vi "手动启动选择对话框.vi"() -> (2 "确定":bool, 3 "输出簇":T1)   [LabVIEW 2016, in "PLC.lvlib"]
uses:
  PLC.lvlib
panel:
  in  "总磷":bool
  in  "测试模式":enum16{"正常测试", "集成干预"}(ring)
  in  "CODCr":bool
  in  "总氮":bool
  in  "氨氮":bool
  in  "CODmn":bool
  in  "多参数":bool
  in  "取消":bool
  in  "确定":bool
  # "请选择启动参数"
  # "请选择启动模式："
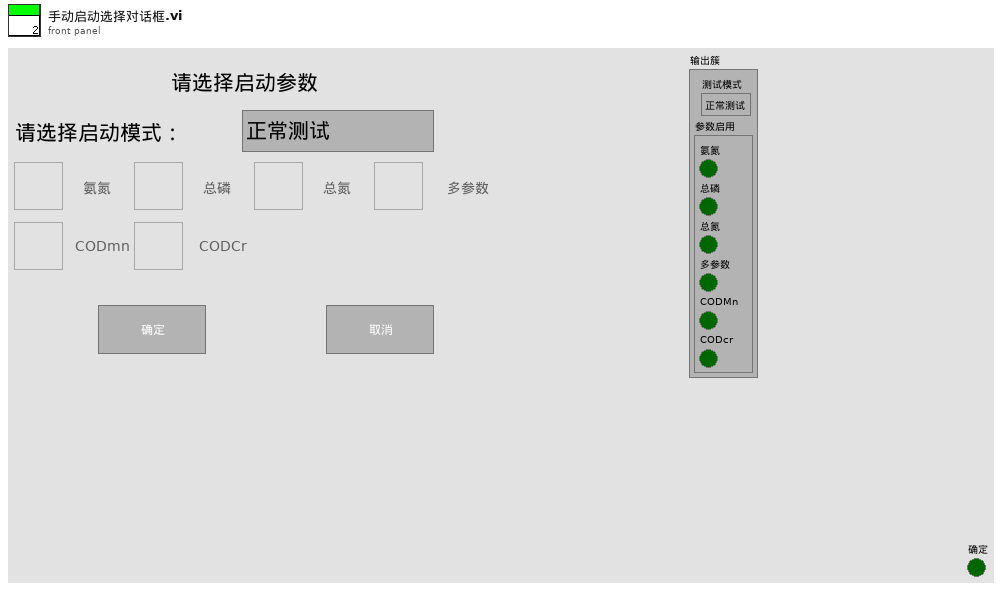
[diagram p1: front panel]
types:
  T1 = cluster{"测试模式":enum16{"正常测试", "集成干预"}, "参数启用":cluster{"氨氮":bool, "总磷":bool, "总氮":bool, "多参数":bool, "CODMn":bool, "CODcr":bool}}
  T2 = enum8{"Enabled", "Disabled", "Disabled and Grayed Out"}
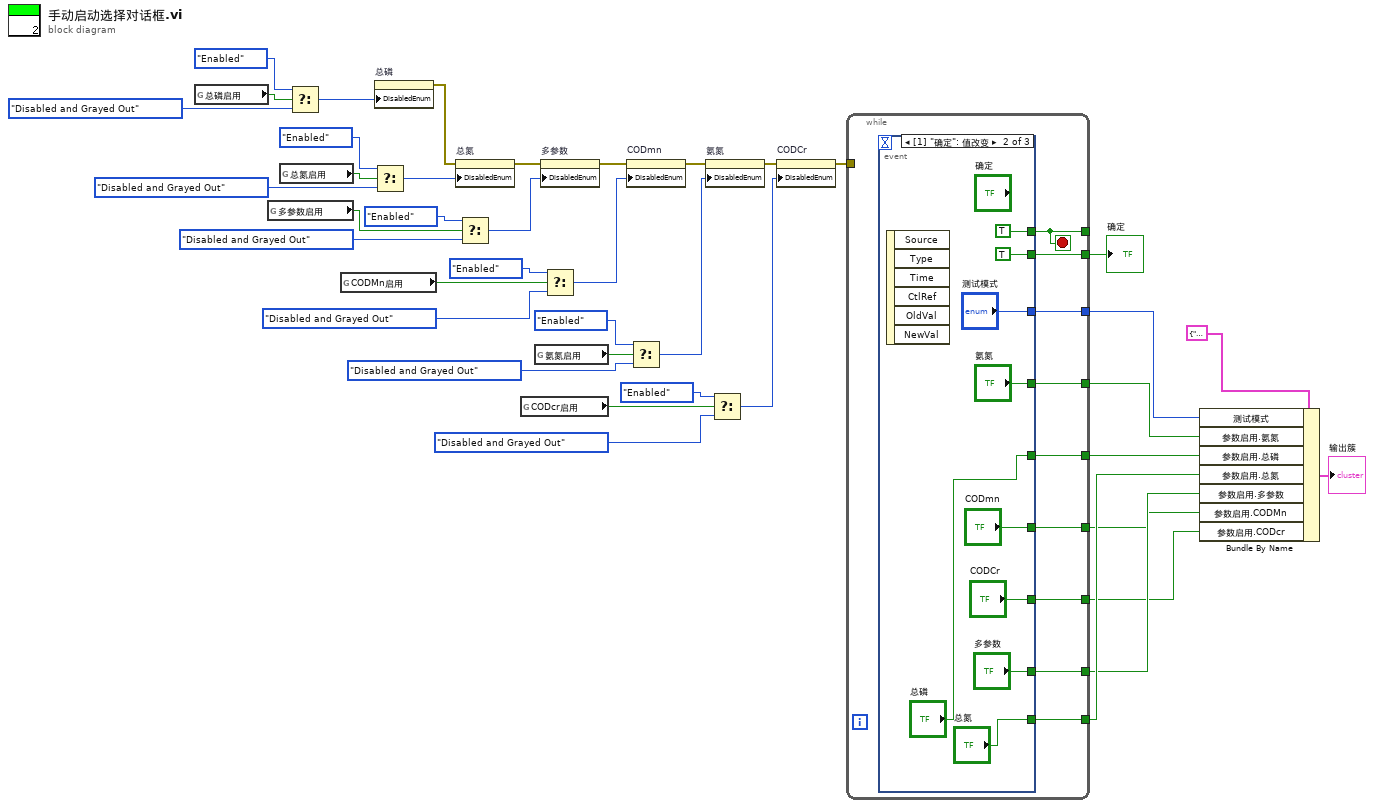
[diagram p0: block diagram]
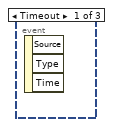
[diagram p2: hidden frame]
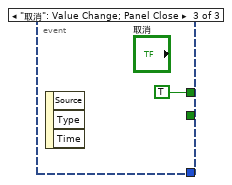
[diagram p3: hidden frame]
diagram:
  n1 = global read "系统设置全局变量.vi" "总磷启用"() -> (w8:bool)
  n2 = global read "系统设置全局变量.vi" "多参数启用"() -> (w21:bool)
  n3 = global read "系统设置全局变量.vi" "总氮启用"() -> (w39:bool)
  n4 = Select(t=T2."Enabled" ("禁用"), s=w8, f=T2."Disabled and Grayed Out" ("禁用")) -> (s? t:f=w11:T2)
  n5 = global read "系统设置全局变量.vi" "CODMn启用"() -> (w25:bool)
  n6 = property on="总磷" class="Bool (严格)"("DisabledEnum"=w11) -> (error out=w7:errorcluster)  [unwired: 2 in, 1 out]
  n7 = Select(t=T2."Enabled" ("禁用"), s=w39, f=T2."Disabled and Grayed Out" ("禁用")) -> (s? t:f=w36:T2)
  n8 = property on="总氮" class="Bool (严格)"(error in=w7, "DisabledEnum"=w36) -> (error out=w19:errorcluster)  [unwired: 1 in, 1 out]
  n9 = Select(t=T2."Enabled" ("禁用"), s=w21, f=T2."Disabled and Grayed Out" ("禁用")) -> (s? t:f=w20:T2)
  n10 = global read "系统设置全局变量.vi" "CODcr启用"() -> (w23:bool)
  n11 = global read "系统设置全局变量.vi" "氨氮启用"() -> (w27:bool)
  n12 = property on="多参数" class="Bool (严格)"(error in=w19, "DisabledEnum"=w20) -> (error out=w18:errorcluster)  [unwired: 1 in, 1 out]
  n13 = Select(t=T2."Enabled" ("禁用"), s=w25, f=T2."Disabled and Grayed Out" ("禁用")) -> (s? t:f=w24:T2)
  n14 = property on="CODmn" class="Bool (严格)"(error in=w18, "DisabledEnum"=w24) -> (error out=w17:errorcluster)  [unwired: 1 in, 1 out]
  n15 = Select(t=T2."Enabled" ("禁用"), s=w27, f=T2."Disabled and Grayed Out" ("禁用")) -> (s? t:f=w26:T2)
  n16 = property on="氨氮" class="Bool (严格)"(error in=w17, "DisabledEnum"=w26) -> (error out=w16:errorcluster)  [unwired: 1 in, 1 out]
  n17 = Select(t=T2."Enabled" ("禁用"), s=w23, f=T2."Disabled and Grayed Out" ("禁用")) -> (s? t:f=w22:T2)
  n18 = property on="CODCr" class="Bool (严格)"(error in=w16, "DisabledEnum"=w22) -> (error out=w15:errorcluster)  [unwired: 1 in, 1 out]
  n19 = while {
    tunnel: [w49] -> w4
    tunnel: [w48] -> w13
    tunnel: [w47] -> w3
    tunnel: [w46] -> _
    tunnel: [w45] -> w40
    tunnel: [w44] -> w12
    tunnel: [w43] -> w2
    tunnel: w15 -> [_]
    tunnel: [w42] -> w14
    tunnel: [w41] -> w5
    stop <- w46 stop-if-true
    n20 = event shown="[1] \"确定\": 值改变" {
      selector: _ -> [_ _ _]
      dyn-events: _ -> [_ _ _]
      timeout: _ -> [_ _ _]
      tunnel: [_ TRUE TRUE] -> w46
      tunnel: [_ "多参数" _] -> w49
      tunnel: [_ "氨氮" _] -> w48
      tunnel: [_ "CODmn" _] -> w47
      tunnel: [_ TRUE _] -> w45
      tunnel: [_ "总磷" _] -> w44
      tunnel: [_ "CODCr" _] -> w43
      tunnel: [_ "测试模式" _] -> w42
      tunnel: [_ "总氮" _] -> w41
      event Timeout {
        n21 = event-data() -> ()  [unwired: 1 in, 3 out]
      }
      event "确定": Value Change {
        n22 = event-data() -> ()  [unwired: 1 in, 6 out]
      }
      event "取消": Value Change; Panel Close {
        n23 = event-data() -> ()  [unwired: 1 in, 3 out]
      }
    }
  }
  "确定" <- w40
  n24 = Bundle By Name(cluster=T1 {"测试模式"=enum."正常测试", "参数启用"={"氨氮"=FALSE, "总磷"=FALSE, "总氮"=FALSE, "多参数"=FALSE, "CODMn"=FALSE, "CODcr"=FALSE}} ("参数"), "测试模式"=w14, "参数启用.氨氮"=w13, "参数启用.总磷"=w12, "参数启用.总氮"=w5, "参数启用.多参数"=w4, "参数启用.CODMn"=w3, "参数启用.CODcr"=w2) -> (→"输出簇":T1)
